vi "indexer commands (SubVI).vi"(10 "SPEED":dbl, 11 "ACCELERATION":dbl) -> (2 "String":string, 3 "String 2":string)   [LabVIEW 2015]
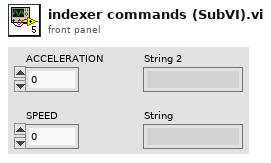
[diagram p1: front panel]
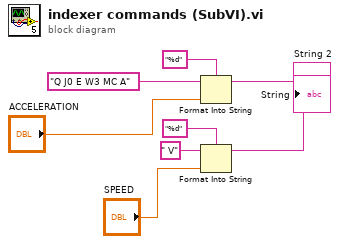
[diagram p0: block diagram]
diagram:
  n1 = Format Into String(format string="%d", initial string="Q J0 E W3 MC A", "ACCELERATION") -> (resulting string=→"String 2":string)  [unwired: 1 in, 1 out]
  n2 = Format Into String(format string="%d", initial string=" V", "SPEED") -> (resulting string=→"String":string)  [unwired: 1 in, 1 out]
